vi "Message Handling Daemon.vi"(1 "message event":refnum<user-event>, 2 "message queue":refnum<queue>) -> ()   [LabVIEW 2018]
uses:
  Classes/Message/Message.lvclass
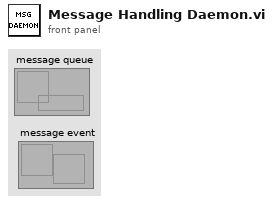
[diagram p1: front panel]
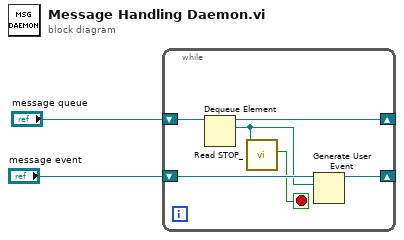
[diagram p0: block diagram]
diagram:
  n1 = while {
    shift-right: [w3] -> _
    shift-left: "message queue" -> [w8]
    shift-right: [w4] -> _
    shift-left: "message event" -> [w7]
    stop <- w6 stop-if-true
    n2 = Dequeue Element(queue=w8) -> (queue out=w3:refnum<queue>, element=w5:refnum<class "Message.lvclass">)  [unwired: 2 in, 2 out]
    n3 = call-dynamic "Read STOP_.vi"("Message in"=w5) -> ("STOP?"=w6:bool)  [unwired: 8 in, 2 out]
    n4 = Generate User Event(user event=w7, event data cluster=w5) -> (user event out=w4:refnum<user-event>)  [unwired: 2 in, 1 out]
  }
